vi "Debug.vi"(10 "Method":string, 11 "jettl Queue Actor in":refnum<class "jettl Queue Actor.lvclass">) -> (3 "jettl Queue Actor out":refnum<class "jettl Queue Actor.lvclass">)   [LabVIEW 2021, in "jettl.lvlib" / "jettl Queue Actor.lvlib" / "jettl Queue Actor.lvclass"]
uses:
  jettl Queue Actor.lvclass
  jettl Queue Actor.lvclass/jettl Queue Actor.ctl
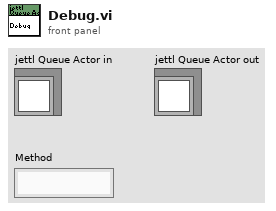
[diagram p1: front panel]
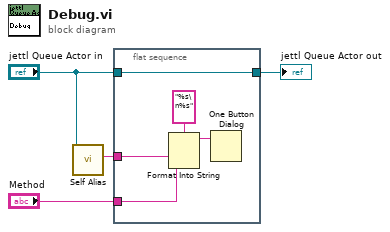
[diagram p0: block diagram]
diagram:
  n1 = call-dynamic "Self Alias.vi"("jettl Queue Actor in"="jettl Queue Actor in") -> ("Self Alias"=w2:string)  [unwired: 10 in]
  n2 = flat-sequence {
    tunnel: [w9] -> w4
    tunnel: "jettl Queue Actor in" -> [w9]
    tunnel: "Method" -> [w5]
    tunnel: w2 -> [w6]
    frame #0 {
      n3 = Format Into String(format string="%s\n%s", w6, w5) -> (resulting string=w7:string)  [unwired: 2 in, 1 out]
      n4 = One Button Dialog(message=w7) -> ()  [unwired: 1 in, 1 out]
    }
  }
  "jettl Queue Actor out" <- w4
